vi "init.vi"(8 "error in":errorcluster, 10 "TBM module configuration in":refnum<class "TBM module configuration.lvclass">, 11 "TDMS datalogger runtime in":refnum<class "TDMS datalogger runtime.lvclass">) -> (0 "error out":errorcluster, 1 "data allocations":T1, 2 "execution settings":T4, 3 "TDMS datalogger runtime out":refnum<class "TDMS datalogger runtime.lvclass">)   [LabVIEW 2013, in "TDMS datalogger runtime.lvclass"]
doc: "Provides an interface for initializing a module at runtime. While this interface performs no operations, a child should provide an override which may open any necessary references or sessions, allocate necessary memory, and perform any final configuration validataion before providing the full configuration <b>execution data</b> to the calling process."
uses:
  TDMS datalogger runtime.lvclass
  <vilib>/NI/Tag Bus Module Framework/module configuration/TBM module configuration.lvclass
  <vilib>/NI/Tag Bus Module Framework/runtime/execution settings.ctl
  <vilib>/NI/Tag Bus Module Framework/channel/data tables.ctl
  <vilib>/NI/Tag Bus/dictionary/data dictionary.lvclass
  <vilib>/NI/Tag Bus/dictionary table pair.ctl
  <vilib>/NI/Tag Bus/table/data table.ctl
  configuration/TDMS datalogger configuration.lvclass
  message to background process.ctl
  control enum.ctl
  response from background process.ctl
  response enum.ctl
  configuration/TDMS datalogger configuration.lvclass/TDMS datalogger configuration.ctl
  <vilib>/NI/Configuration Framework/serializable configuration/NISE_CEF_serializable configuration.lvclass/NISE_CEF_serializable configuration.ctl
  TDMS datalogger runtime.lvclass/TDMS datalogger runtime.ctl
  configuration/Read add enable channel.vi
  <vilib>/NI/Configuration Framework/serializable configuration/Read UID.vi
  configuration/Read queue size.vi
  configuration/Read Path.vi
  configuration/Read backup directory.vi
  configuration/Read scans per write.vi
  configuration/Read log name.vi
  configuration/Read logrotate_options.vi
  <vilib>/Utility/LVClass/Get LV Class Name.vi
  <vilib>/NI/Configuration Framework/error generator/NISE_error generator.vi
  <vilib>/NI/Tag Bus Module Framework/channel/TBM channel.lvclass
  <vilib>/NI/Tag Bus Module Framework/runtime/TBM module execution interface.lvclass
  <vilib>/NI/Tag Bus/table/data table.lvlib
  <vilib>/NI/LogRotate/LogRotate.lvclass
  <vilib>/NI/Tag Bus/tag bus.lvlib
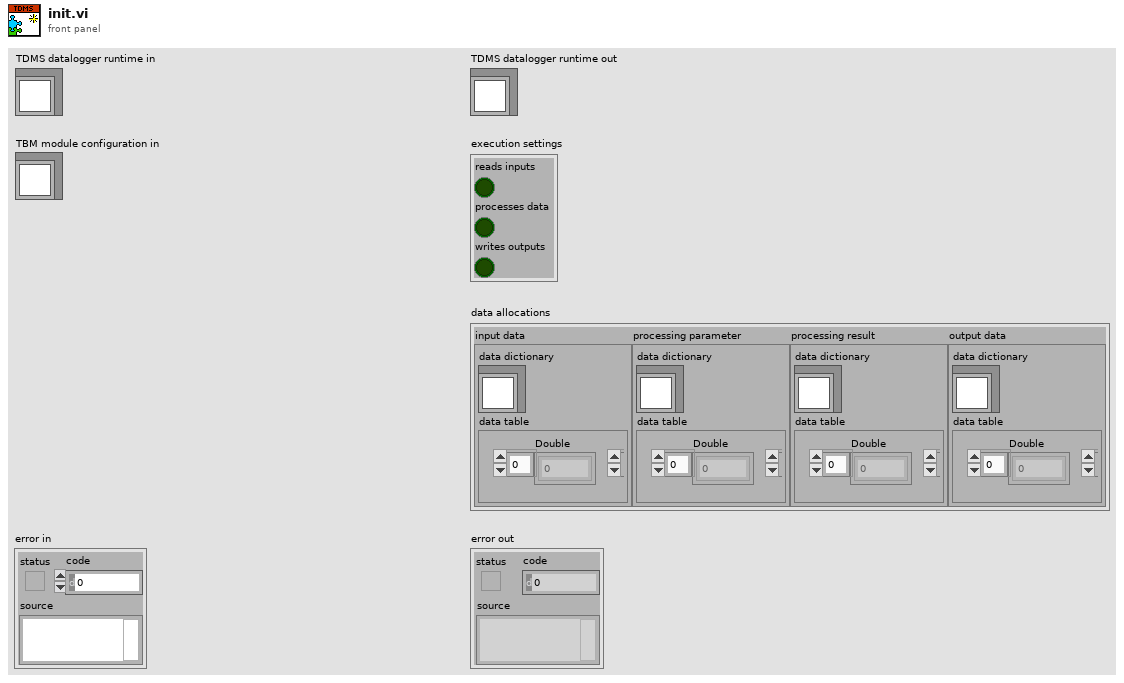
[diagram p1: front panel]
types:
  T1 = typedef "TBM channel.lvclass/data tables.ctl" = cluster{"input data":T2, "processing parameter":T2, "processing result":T2, "output data":T2}
  T2 = typedef "tag bus.lvlib/dictionary table pair.ctl" = cluster{"data dictionary":refnum<class "data dictionary.lvclass">, "data table":T3}
  T3 = typedef "tag bus.lvlib/data table.lvlib/data table.ctl" = cluster{"Double":dbl[], "Single":sgl[], "I64":i64[], "I32":i32[], "I16":i16[], "I8":i8[], "U64":u64[], "U32":u32[], "U16":u16[], "U8":u8[], "Boolean":bool[], "String":string[], "Array of Double":cluster{"DBL Array":dbl[]}[], "Array of Single":cluster{"SGL Array":sgl[]}[], "Array of I64":cluster{"I64 Array":i64[]}[], "Array of I32":cluster{"I32 Array":i32[]}[], "Array of I16":cluster{"I16 Array":i16[]}[], "Array of I8":cluster{"I8 Array":i8[]}[], "Array of U64":cluster{"U64 Array":u64[]}[], "Array of U32":cluster{"U32 Array":u32[]}[], "Array of U16":cluster{"U16 Array":u16[]}[], "Array of U8":cluster{"U8 Array":u8[]}[], "Array of Boolean":cluster{"Boolean Array":bool[]}[], "Array of String":cluster{"String Array":string[]}[]}
  T4 = typedef "TBM module execution interface.lvclass/execution settings.ctl" = cluster{"reads inputs":bool, "processes data":bool, "writes outputs":bool}
  T5 = cluster{"read mode":enum16{"polling", "blocking"}, "write mode":enum16{"polling", "blocking"}}
  T6 = typedef "TDMS datalogger runtime.lvclass/response from background process.ctl" = cluster{"response enum":T7, "datapack":refnum<data-value>, "error code":i32}
  T7 = typedef "TDMS datalogger runtime.lvclass/response enum.ctl" = enum16{"exit", "return buffer", "error"}
  T8 = typedef "TDMS datalogger runtime.lvclass/message to background process.ctl" = cluster{"control enum":T9, "datapack":refnum<data-value>, "Time Stamp":timestamp}
  T9 = typedef "TDMS datalogger runtime.lvclass/control enum.ctl" = enum16{"exit", "output data"}
  T10 = typedef "tag bus.lvlib/tag descriptor.lvclass/Data Type.ctl" = enum16{"Double", "Single", "I64", "I32", "I16", "I8", "U64", "U32", "U16", "U8", "Boolean", "String", "Array of Double", "Array of Single", "Array of I64", "Array of I32", "Array of I16", "Array of I8", "Array of U64", "Array of U32", "Array of U16", "Array of U8", "Array of Boolean", "Array of String"}
  T11 = typedef "LogRotate.lvclass/options.ctl" = cluster{"max file size (bytes)":i64, "rotate count":u32, "max age (days)":dbl, "No archive dir":bool, "Archive dir":path}
  T12 = typedef "tag bus.lvlib/data dictionary.lvclass/full data dictionary.ctl" = cluster{"Double":string[], "Single":string[], "I64":string[], "I32":string[], "I16":string[], "I8":string[], "U64":string[], "U32":string[], "U16":string[], "U8":string[], "Boolean":string[], "String":string[], "Array of Double":string[], "Array of Single":string[], "Array of I64":string[], "Array of I32":string[], "Array of I16":string[], "Array of I8":string[], "Array of U64":string[], "Array of U32":string[], "Array of U16":string[], "Array of U8":string[], "Array of Boolean":string[], "Array of String":string[]}
  T13 = typedef "tag bus.lvlib/data table.lvlib/allocation specification.ctl" = cluster{"data type":T10, "size":i32}
  T14 = typedef "TDMS datalogger runtime.lvclass/data cache.ctl" = cluster{"timestamps":timestamp[], "Double":dbl[][], "Single":sgl[][], "I64":i64[][], "I32":i32[][], "I16":i16[][], "I8":i8[][], "U64":u64[][], "U32":u32[][], "U16":u16[][], "U8":u8[][], "Boolean":bool[][]}
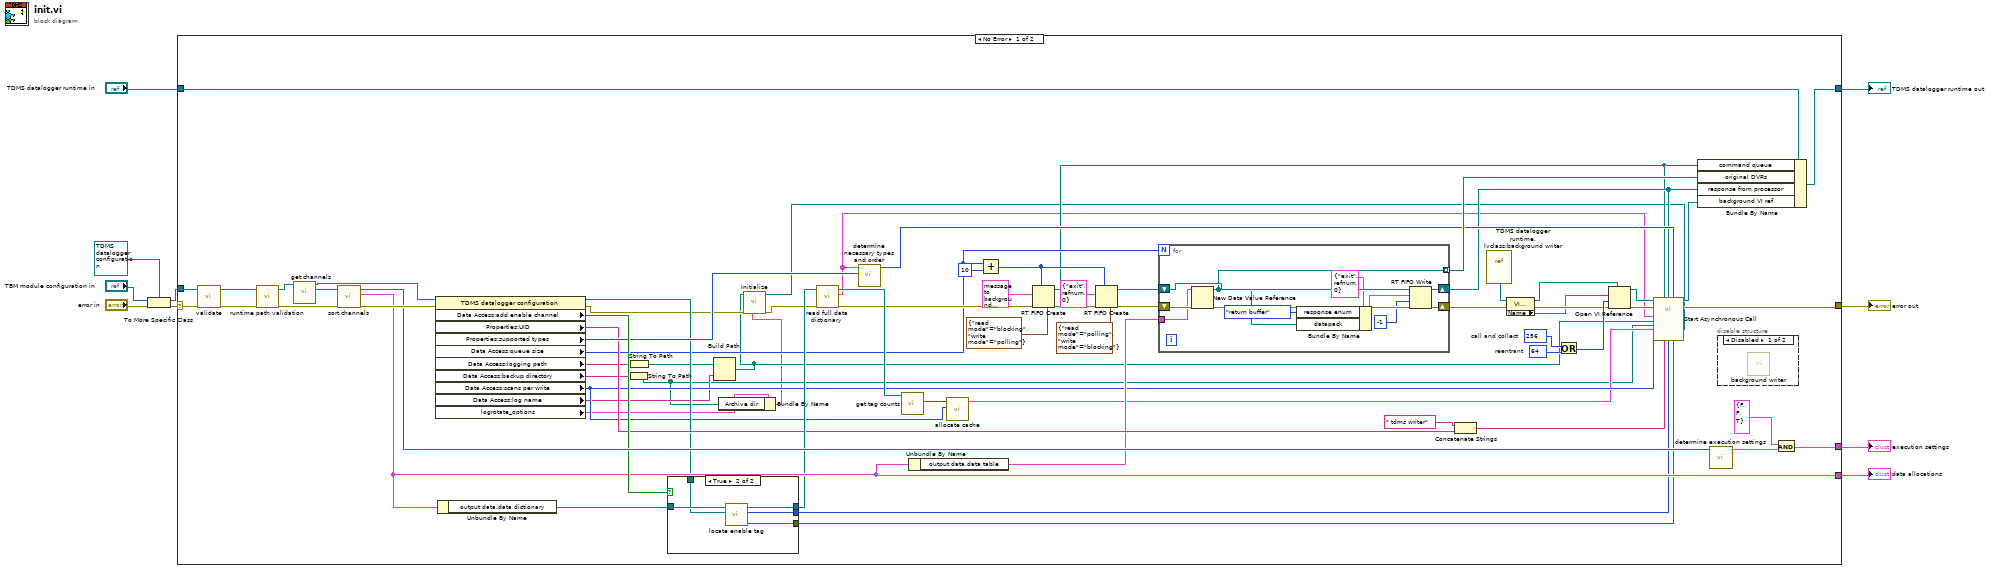
[diagram p0: block diagram]
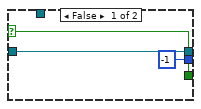
[diagram p2: hidden frame]
diagram:
  n1 = To More Specific Class(target class=refnum<class "TDMS datalogger configuration.lvclass"> refnum ("Synchronous module configuration"), reference="TBM module configuration in", error in="error in") -> (specific class reference=w9:refnum<class "TDMS datalogger configuration.lvclass">, error out=w10:errorcluster)
  n2 = case shown="No Error" w10 {
    selector: w10 -> [w76 w100]
    tunnel: w9 -> [w75 _]
    tunnel: "TDMS datalogger runtime in" -> [w74 w101]
    tunnel: [w73 w101] -> w4
    tunnel: [w62 w100] -> w3
    tunnel: [w59 _] -> w1
    tunnel: [w72 _] -> w2
    frame No Error {
      w67 = 64  # reentrant
      w66 = 256  # call and collect
      n3 = call-dynamic "validate.vi"("error in"=w76, "TDMS datalogger configuration in"=w75) -> ("error out"=w77:errorcluster, "TDMS datalogger configuration out"=w51:refnum<class "TDMS datalogger configuration.lvclass">)  [unwired: 8 in]
      n4 = call "runtime path validation.vi"("error in"=w77, "TDMS datalogger configuration in"=w51) -> ("error out"=w52:errorcluster, "TDMS datalogger configuration out"=w50:refnum<class "TDMS datalogger configuration.lvclass">)  [unwired: 8 in]
      n5 = call-dynamic "get channels.vi"("module configuration in"=w50) -> ("channels"=w48:refnum<class "TBM channel.lvclass">[], "module configuration out"=w49:refnum<class "TDMS datalogger configuration.lvclass">)  [unwired: 9 in]
      n6 = call <vilib>:"sort channels.vi"("error in"=w52, "channels in"=w48) -> ("error out"=w80:errorcluster, "data allocations"=w59:T1, "channels out"=w78:refnum<class "TBM channel.lvclass">[])  [unwired: 7 in]
      n7 = property class="TDMS datalogger configuration"(reference=w49, error in=w80) -> (reference out=w44:refnum<class "TDMS datalogger configuration.lvclass">, error out=w17:errorcluster, "Data Access:add enable channel"=w60:bool, "Properties:UID"=w54:string, "Properties:supported types"=w55:T10[], "Data Access:queue size"=w36:u16, "Data Access:logging path"=w21:string, "Data Access:backup directory"=w20:string, "Data Access:scans per write"=w27:u16, "Data Access:log name"=w19:string, "logrotate_options"=w15:T11)
      n8 = Unbundle By Name(w59) -> ("output data.data dictionary"=w61:refnum<class "data dictionary.lvclass">)
      n9 = String To Path(string=w20) -> (path=w14:path)
      n10 = String To Path(string=w21) -> (path=w18:path)
      n11 = case shown="True" w60 {
        selector: w60 -> [w83 _]
        tunnel: w61 -> [w82 w88]
        tunnel: [w82 w87] -> w57
        tunnel: [w83 w85] -> w30
        tunnel: [-1 ("index") w86] -> w29
        tunnel: w44 -> [_ w84]
        frame False {
        }
        frame True {
          n12 = call "locate enable tag.vi"("TDMS datalogger configuration"=w84, "data dictionary in"=w88) -> ("found?"=w85:bool, "index"=w86:i32, "data dictionary out"=w87:refnum<class "data dictionary.lvclass">)  [unwired: 7 in]
        }
      }
      n13 = Build Path(base path=w18, name or relative path=w19) -> (appended path=w16:path)
      n14 = Bundle By Name(cluster=w15, "Archive dir"=w14) -> (w13:T11)
      n15 = call <vilib>:"Initialize.vi"("Options"=w13, "error in (no error)"=w17, "Log File Path"=w16) -> ("error out"=w12:errorcluster, "LogRotate"=w11:refnum<class "LogRotate.lvclass">)  [unwired: 7 in]
      n16 = call <vilib>:"read full data dictionary.vi"("error in"=w12, "data dictionary in"=w57) -> ("error out"=w46:errorcluster, "dictionary"=w22:T12, "data dictionary out"=w56:refnum<class "data dictionary.lvclass">)  [unwired: 7 in]
      n17 = call "determine necessary types and order.vi"("supported types"=w55, "dictionary"=w22) -> ("output type order"=w25:T10[])  [unwired: 9 in]
      n18 = call <vilib>:"get tag counts.vi"("data dictionary in"=w56) -> ("counts"=w70:T13[])  [unwired: 9 in, 1 out]
      n19 = Unbundle By Name(w59) -> ("output data.data table"=w47:T3)
      n20 = call "allocate cache.vi"("scans per write"=w27, "counts"=w70) -> ("cache allocation"=w26:T14)  [unwired: 9 in]
      n21 = Add(x=w36, y=u16 10) -> (x+y=w34:u16)
      n22 = RT FIFO Create(1:T8 {"control enum"=enum."exit", "datapack"=refnum, "Time Stamp"=timestamp(0 s since 1904-01-01)} ("message"), 3:w46, 4:w34, 7:T5 {"read mode"=enum."blocking", "write mode"=enum."polling"} ("r/w modes (polling,polling)")) -> (8:w23:refnum<k33>, 11:w45:errorcluster)  [unwired: 4 in, 1 out]
      n23 = RT FIFO Create(1:T6 {"response enum"=enum."exit", "datapack"=refnum, "error code"=0} ("message"), 3:w45, 4:w34, 7:T5 {"read mode"=enum."polling", "write mode"=enum."blocking"} ("r/w modes (polling,polling)")) -> (8:w37:refnum<k33>, 11:w41:errorcluster)  [unwired: 4 in, 1 out]
      n24 = for {
        N: w36 -> [_]
        shift-right: [w96] -> w63
        shift-left: w41 -> [w99]
        tunnel: w47 -> [w98]
        tunnel: [w90] -> w38 mode=indexing
        shift-right: [w95] -> w24
        shift-left: w37 -> [w94]
        n25 = New Data Value Reference(data value=w98, error in=w99) -> (data value reference=w90:refnum<data-value>, error out=w97:errorcluster)
        n26 = Bundle By Name(cluster=T6 {"response enum"=enum."exit", "datapack"=refnum, "error code"=0} ("element"), "response enum"=response_enum."return buffer", "datapack"=w90) -> (w91:T6)
        n27 = RT FIFO Write(0:w94, 1:w91, 2:-1 ("timeout in ms (0)"), 3:w97) -> (8:w95:refnum<k33>, 11:w96:errorcluster)  [unwired: 1 in, 2 out]
      }
      n28 = Concatenate Strings(" tdms writer" ("string"), w54) -> (w28:string)
      n29 = vi-ref "TDMS datalogger runtime.lvclass:background writer.vi"() -> (w33:refnum<vi>)
      n30 = property class="VI (strict)"(reference=w33, error in=w63) -> (reference out=w32:refnum<vi>, error out=w65:errorcluster, "Name"=w64:string)
      n31 = Or(x=w66, y=w67) -> (x .or. y?=w68:i32)
      n32 = Open VI Reference(type specifier VI Refnum (for type only)=w32, vi path=w64, options=w68, error in (no error)=w65) -> (vi reference=w31:refnum<vi>, error out=w69:errorcluster)  [unwired: 2 in]
      n33 = call-by-ref "Start Asynchronous Call"(reference=w31, error in=w69, "dictionary"=w22, "command queue"=w23, "response from processor"=w24, "output type order"=w25, "logging path"=w16, "backup directory"=w14, "cache allocation"=w26, "LogRotate"=w11, "scans per write"=w27, "group name"=w28, "enable channel (bool)"=w29, "has enable channel"=w30) -> (reference out=w58:refnum<vi>, error out=w62:errorcluster)  [unwired: 3 in, 1 out]
      n34 = Bundle By Name(cluster=w74, "command queue"=w23, "original DVRs"=w38, "response from processor"=w24, "background VI ref"=w58) -> (w73:refnum<class "TDMS datalogger runtime.lvclass">)
      n35 = call <vilib>:"determine execution settings.vi"("channels"=w78) -> ("execution settings"=w79:T4)  [unwired: 10 in]
      n36 = disable-structure shown="Disabled" {
        frame Disabled {
          n37 = call "background writer.vi"() -> ()  [unwired: 15 in, 1 out]
        }
        frame Enabled {
        }
      }
      n38 = And(x=T4 {"reads inputs"=FALSE, "processes data"=FALSE, "writes outputs"=TRUE}, y=w79) -> (x .and. y?=w72:T4)
    }
    frame Error {
    }
  }
  "error out" <- w3
  "TDMS datalogger runtime out" <- w4
  "execution settings" <- w2
  "data allocations" <- w1
